vi "emi_Splash Update.vi"(9 "error In":errorcluster, 13 "Task Text":string) -> (10 "error out":errorcluster)   [LabVIEW 2011]
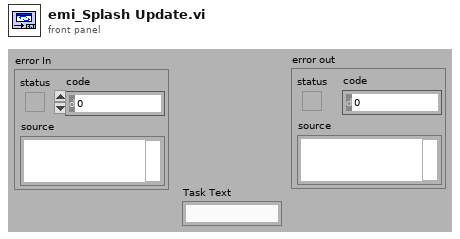
[diagram p1: front panel]
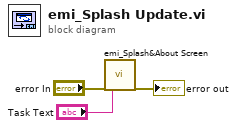
[diagram p0: block diagram]
diagram:
  n1 = call "emi_Splash&About Screen.vi"("error in (no error)"="error In", "Status text"="Task Text") -> ("error out"=→"error out":errorcluster)  [unwired: 17 in]
